vi "Day1-a.vi"(10 "Input":string="15931\n8782\n16940\n14614\n\n4829\n12415\n13259\n11441\n8199\n\n2540\n2500\n6341\n2235\n1858\n4157\n5053\n6611\n1050\n4401\n6187\n1078\n3297\n\n25264\n23014\n15952\n\n10156\n4544\n4930\n11786\n15822\n\n1264\n6399\n2031\n6892\n3115\n5151\n5093\n6724\n7001\n4011\n1458\n1945\n\n2106\n2016\n1528\n2524\n6089\n4466\n3154\n2686\n3289\n5831\n1520\n2122\n5744\n\n33066\n22616\n\n1993\n8485\n1037\n9730\n2076\n7492\n10000\n2971\n\n11027\n9137\n4599\n7461\n1531\n12939\n\n17530\n18837\n19466\n4845\n\n1467\n4870\n10176\n6657\n5608\n2096\n9977\n6478\n\n18828\n26577\n\n17901\n5059\n13789\n4993\n\n6676\n3415\n2464\n5937\n4275\n6629\n7566\n1943\n6313\n4572\n\n9121\n10713\n5071\n1669\n7736\n10522\n6231\n\n6400\n1771\n4568\n7681\n7486\n60...") -> (2 "Output":i32)   [LabVIEW 2017]
uses:
  OOP/Elf/Elf.lvclass
  OOP/Elf/Elf.lvclass/Elf.ctl
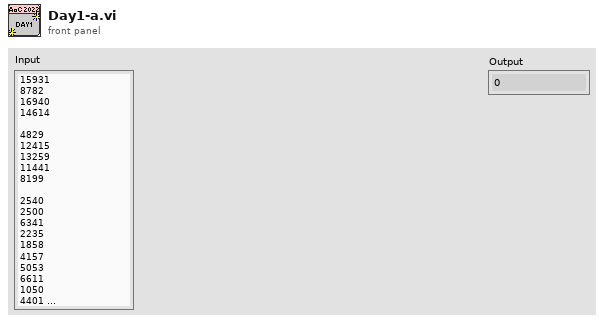
[diagram p1: front panel]
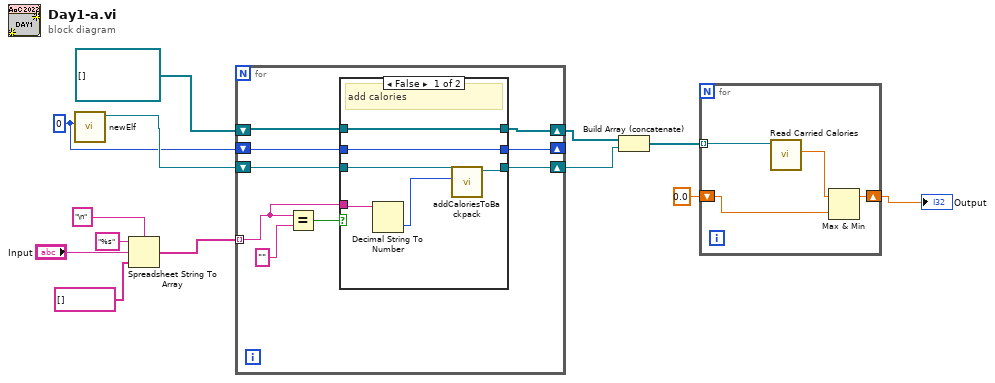
[diagram p0: block diagram]
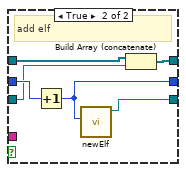
[diagram p2: hidden frame]
diagram:
  w7 = 0 ("Index")
  n1 = call "newElf.vi"("Index"=w7) -> ("Elf out"=w8:refnum<class "Elf.lvclass">)  [unwired: 9 in, 1 out]
  n2 = Spreadsheet String To Array(delimiter (Tab)="\n", format string="%s", spreadsheet string="Input", array type (2D Dbl)=string[] []) -> (array=w10:string[])
  n3 = for {
    tunnel: w10 -> [w14] mode=indexing
    shift-right: [w20] -> w5
    shift-left: refnum<class "Elf.lvclass">[] [] -> [w19]
    shift-right: [w17] -> _
    shift-left: w7 -> [w16]
    shift-right: [w15] -> w4
    shift-left: w8 -> [w18]
    n4 = Equal?(x=w14, y="" ("delimiter (Tab)")) -> (x = y?=w21:bool)
    n5 = case shown="False" w21 {
      tunnel: [w28 w30] -> w20
      tunnel: w19 -> [w28 w31]
      tunnel: w18 -> [w26 w29]
      tunnel: [w27 w33] -> w17
      tunnel: w16 -> [w27 w34]
      tunnel: [w25 w32] -> w15
      tunnel: w14 -> [w24 _]
      frame False {
        # "add calories"
        n6 = Decimal String To Number(string=w24) -> (number=w23:i32)  [unwired: 2 in, 1 out]
        n7 = call-dynamic "addCaloriesToBackpack.vi"("Calories"=w23, "Elf in"=w26) -> ("Elf out"=w25:refnum<class "Elf.lvclass">)  [unwired: 8 in, 1 out]
      }
      frame True {
        # "add elf"
        n8 = Increment(x=w34) -> (x+1=w33:i32)
        n9 = call "newElf.vi"("Index"=w33) -> ("Elf out"=w32:refnum<class "Elf.lvclass">)  [unwired: 9 in, 1 out]
        n10 = Build Array (concatenate)(w31, w29) -> (w30:refnum<class "Elf.lvclass">[])
      }
    }
  }
  n11 = Build Array (concatenate)(w5, w4) -> (w3:refnum<class "Elf.lvclass">[])
  n12 = for {
    tunnel: w3 -> [w38] mode=indexing
    shift-right: [w36] -> w1
    shift-left: 0.0 -> [w35]
    n13 = call "Read Carried Calories.vi"("Elf in"=w38) -> ("Carried Calories"=w37:dbl)  [unwired: 8 in, 2 out]
    n14 = Max & Min(x=w37, y=w35) -> (max(x,y)=w36:dbl)  [unwired: 1 out]
  }
  "Output" <- w1
